vi "Random String.vi"(4 "length":i32) -> (1 "random data":string)   [LabVIEW 2016]
doc: "Outputs a <B>random data</B> string of the specified <B>length</B>."
uses:
  <userlib>/_OpenG.lib/numeric/numeric.llb/Random Number Within Range - I32__ogtk.vi
panel:
  # "Copyright © 2006-2017 JKI. All rights reserved.\n\nThis library is provided \"AS IS\" , WITHOUT WARRANTIES OR \nCONDITIONS OF ANY KIND, either express or implied.\n\nJKI -- http://jki.net"
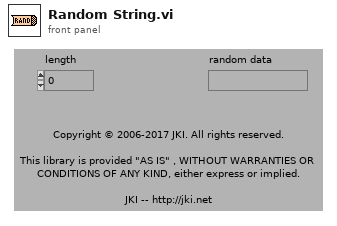
[diagram p1: front panel]
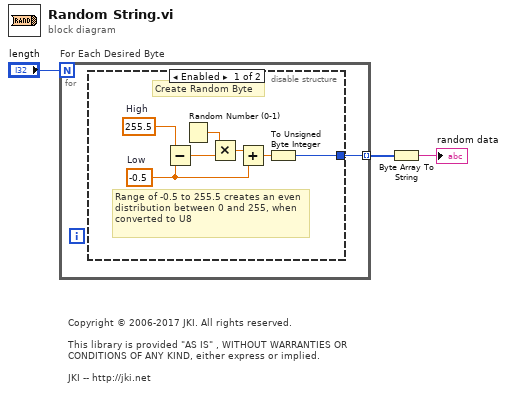
[diagram p0: block diagram]
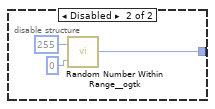
[diagram p2: hidden frame]
diagram:
  # "Copyright © 2006-2017 JKI. All rights reserved.\n\nThis library is provided \"AS IS\" , WITHOUT WARRANTIES OR \nCONDITIONS OF ANY KIND, either express or implied.\n\nJKI -- http://jki.net"
  n1 = for "For Each Desired Byte" {
    N: "length" -> [_]
    tunnel: [w4] -> w2 mode=indexing
    n2 = disable-structure shown="Enabled" {
      disable-tunnel: [w11 w12] -> w4
      frame Enabled {
        w6 = 255.5  # High
        w7 = -0.5  # Low
        # "Range of -0.5 to 255.5 creates an even distribution between 0 and 255, when converted to U8"
        # "Create Random Byte"
        n3 = Subtract(x=w6, y=w7) -> (x-y=w9:dbl)
        n4 = Random Number (0-1)() -> (number: 0 to 1=w8:dbl)
        n5 = Multiply(x=w8, y=w9) -> (x*y=w10:dbl)
        n6 = Add(x=w10, y=w7) -> (x+y=w5:dbl)
        n7 = To Unsigned Byte Integer(number=w5) -> (unsigned 8bit integer=w11:u8)
      }
      frame Disabled {
        n8 = call-poly <userlib>:"Random Number Within Range__ogtk.vi"("High"=u8 255, "Low"=u8 0 ("High")) -> ("Random Number"=w12:i32)  [unwired: 3 in]
      }
    }
  }
  n9 = Byte Array To String(unsigned byte array=w2) -> (string=→"random data":string)
